vi "Sorted Archived Data.vi"(0 "Transactions":T1[](array[typedef])) -> (4 "LBCB 1 \nwith Volts":dbl[](array[numeric]), 6 "LBCB 2\nwith Volts":dbl[](array[numeric]), 8 "LBCB 1":dbl[](array[numeric]), 10 "LBCB 2":dbl[](array[numeric]), 15 "Combined":dbl[](array[numeric]))   [LabVIEW 2013]
uses:
  Transactions/Dataset Source.ctl
  Transactions/Dataset Type.ctl
  Apps/Yes No Button.ctl
  Transactions/Dataset Transaction Id.ctl
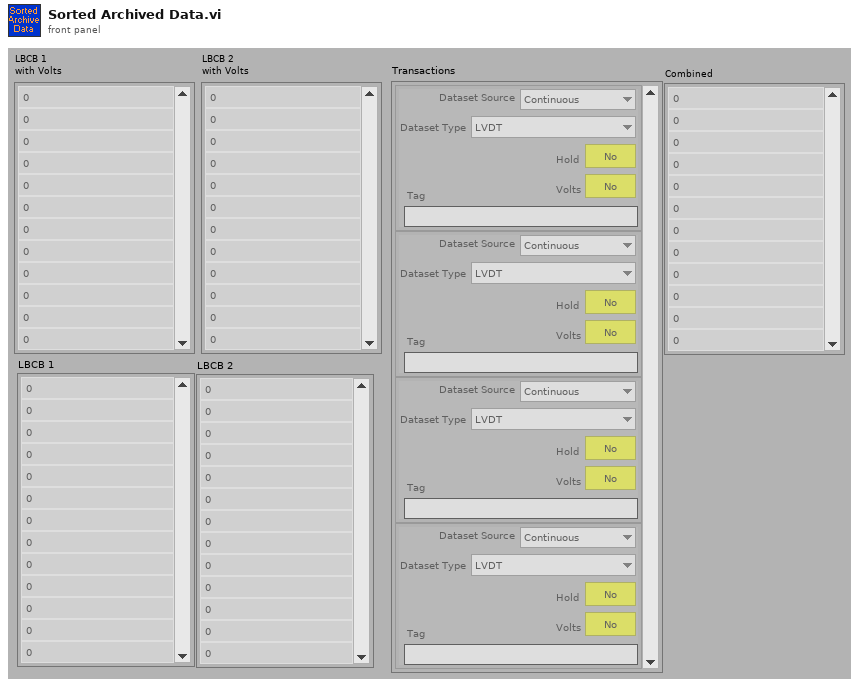
[diagram p1: front panel]
types:
  T1 = typedef "Dataset Transaction Id.ctl" = cluster{"Dataset Source":T2, "Dataset Type":T3, "Hold":T4, "Volts":T4, "Tag":string}
  T2 = typedef "Dataset Source.ctl" = enum16{"Continuous", "Hold", "ED", "Volts", "Offsets", "Increments"}
  T3 = typedef "Dataset Type.ctl" = enum16{"LVDT", "Load Cell", "Actuator Command", "Servo Error", "Displacement Command", "Displacement", "Force"}
  T4 = typedef "Yes No Button.ctl" = bool
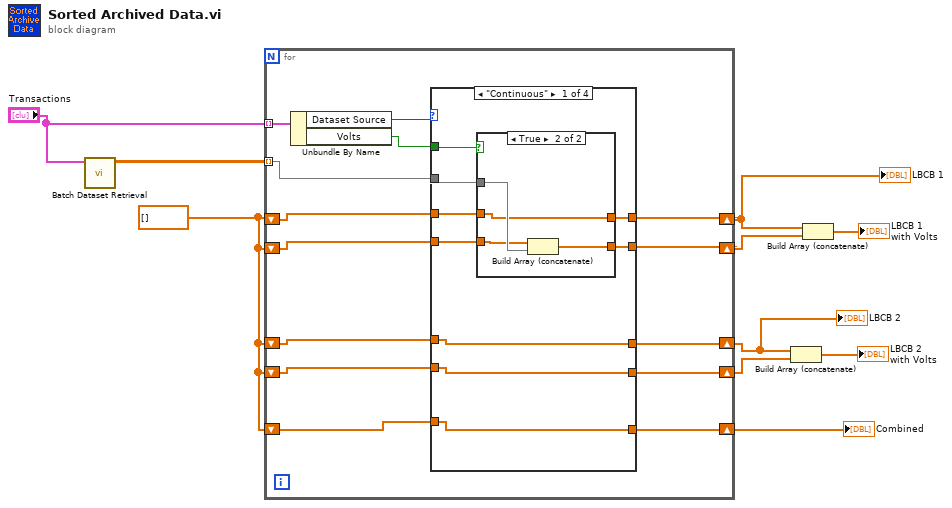
[diagram p0: block diagram]
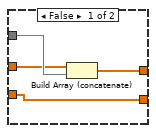
[diagram p2: hidden frame]
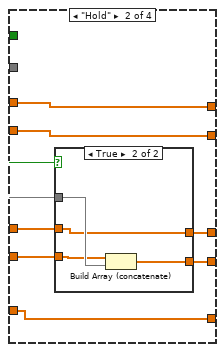
[diagram p3: hidden frame]
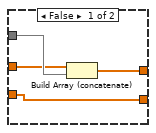
[diagram p4: hidden frame]
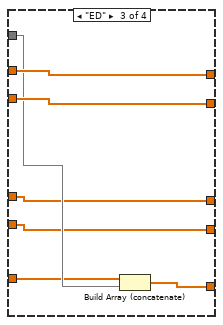
[diagram p5: hidden frame]
diagram:
  w2 = dbl[] []
  n1 = call "Batch Dataset Retrieval.vi"("Transactions"="Transactions") -> ("Data"=w10:dbl[][])  [unwired: 9 in, 1 out]
  n2 = for {
    tunnel: w10 -> [w21] mode=indexing
    tunnel: "Transactions" -> [w24] mode=indexing
    shift-right: [w20] -> w8
    shift-left: w2 -> [w19]
    shift-right: [w18] -> w7
    shift-left: w2 -> [w17]
    shift-right: [w16] -> w1
    shift-left: w2 -> [w14]
    shift-right: [w15] -> w5
    shift-left: w2 -> [w13]
    shift-right: [w12] -> w3
    shift-left: w2 -> [w11]
    n3 = Unbundle By Name(w24) -> ("Dataset Source"=w23:T2, "Volts"=w22:T4)
    n4 = case shown="\"Continuous\"" w23 {
      tunnel: w22 -> [w33 w50 _ _]
      tunnel: w21 -> [w32 w49 w63 _]
      tunnel: [w31 w43 w64 w69] -> w20
      tunnel: w19 -> [w30 w43 w64 w69]
      tunnel: [w29 w44 w65 w70] -> w18
      tunnel: w17 -> [w28 w44 w65 w70]
      tunnel: [w27 w48 w60 w66] -> w16
      tunnel: [w26 w47 w59 w67] -> w15
      tunnel: w14 -> [w27 w46 w60 w66]
      tunnel: w13 -> [w26 w45 w59 w67]
      tunnel: [w25 w42 w62 w68] -> w12
      tunnel: w11 -> [w25 w42 w61 w68]
      frame "Continuous" {
        n5 = case shown="True" w33 {
          tunnel: w32 -> [w36 w41]
          tunnel: [w37 w40] -> w31
          tunnel: w30 -> [w37 w39]
          tunnel: [w35 w38] -> w29
          tunnel: w28 -> [w34 w38]
          frame False {
            n6 = Build Array (concatenate)(w34, w36) -> (w35:dbl[])
          }
          frame True {
            n7 = Build Array (concatenate)(w39, w41) -> (w40:dbl[])
          }
        }
      }
      frame "Hold" {
        n8 = case shown="True" w50 {
          tunnel: w49 -> [w53 w58]
          tunnel: [w54 w57] -> w47
          tunnel: w45 -> [w54 w56]
          tunnel: [w52 w55] -> w48
          tunnel: w46 -> [w51 w55]
          frame False {
            n9 = Build Array (concatenate)(w51, w53) -> (w52:dbl[])
          }
          frame True {
            n10 = Build Array (concatenate)(w56, w58) -> (w57:dbl[])
          }
        }
      }
      frame "ED" {
        n11 = Build Array (concatenate)(w61, w63) -> (w62:dbl[])
      }
      frame "Volts" {
      }
    }
  }
  "Combined" <- w3
  "LBCB 1" <- w7
  "LBCB 2" <- w1
  n12 = Build Array (concatenate)(w1, w5) -> (→"LBCB 2\nwith Volts":dbl[])
  n13 = Build Array (concatenate)(w7, w8) -> (→"LBCB 1 \nwith Volts":dbl[])
